vi "usrp set gpio attr.vi"(5 "mboard":u64, 6 "mask":u32, 7 "value":u32, 8 "error in (no error)":errorcluster, 9 "attr":string, 10 "bank":string, 11 "h":u64) -> (0 "error out":errorcluster, 3 "function return":u32(ring))   [LabVIEW 2023, in "uhd.lvlib"]
doc: "UHD_API uhd_error uhd_usrp_set_gpio_attr(uhd_usrp_handle h,\n const char* bank,\n const char* attr,\n uint32_t value,\n uint32_t mask,\n size_t mboard);"
uses:
  <userlib>/uhd/uhd.lvlib
  <userlib>/uhd/uhd.dll
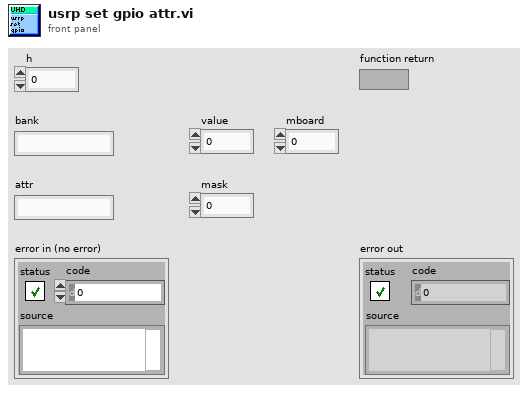
[diagram p1: front panel]
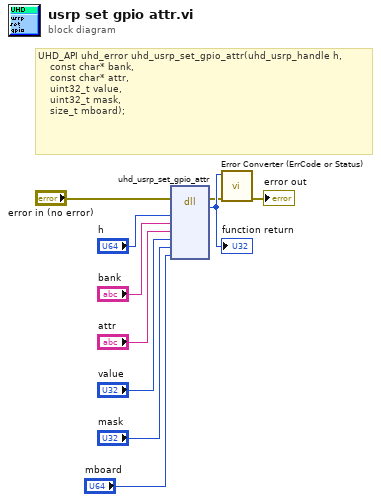
[diagram p0: block diagram]
diagram:
  # "UHD_API uhd_error uhd_usrp_set_gpio_attr(uhd_usrp_handle h,\n    const char* bank,\n    const char* attr,\n    uint32_t value,\n    uint32_t mask,\n    size_t mboard);"
  n1 = dll-call lib="C:/Program Files/National Instruments/LabVIEW 2023/user.lib/uhd/uhd.*" fn="uhd_usrp_set_gpio_attr"(error in="error in (no error)", "h"="h", "bank"="bank", "attr"="attr", "value"="value", "mask"="mask", "mboard"="mboard") -> (error out=w2:errorcluster, w10:u32)  [unwired: 8 in, 1 out]
  "function return" <- w10
  n2 = call <userlib>:"Error Converter (ErrCode or Status).vi"("error in (no error)"=w2, "error code"=w10) -> ("error out"=→"error out":errorcluster)  [unwired: 9 in]
